vi "Init.vi"(8 "Error In":errorcluster, 11 "Communicator in":refnum<class "Communicator.lvclass">) -> (0 "Error Out":errorcluster, 3 "Communicator out":refnum<class "Communicator.lvclass">)   [LabVIEW 2019, in "Communicator.lvclass"]
uses:
  Communicator.lvclass
  Interfaces/IConfigure/IConfigure.lvclass
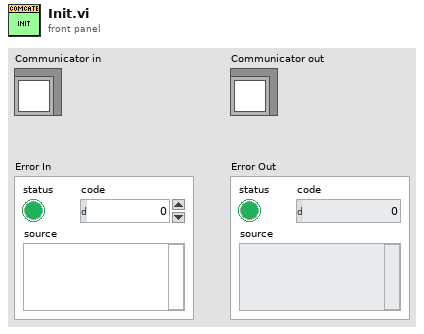
[diagram p1: front panel]
types:
  T1 = typedef "Communicator.lvclass/ObjectAttributes.ctl" = cluster{"IConfigure":refnum<class "IConfigure.lvclass">, "Worker Enqueuer":refnum<class "Message Enqueuer.lvclass">, "Start Counter":i32, "Msg Sent":refnum<user-event>}
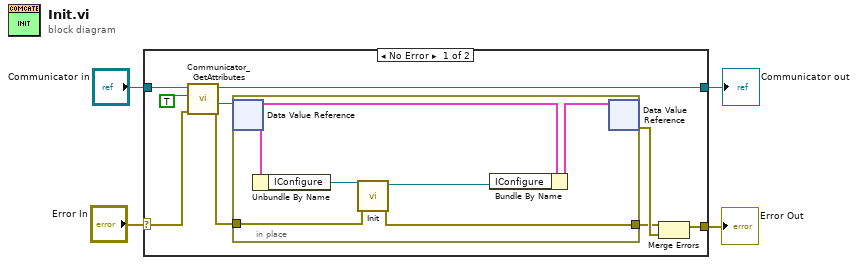
[diagram p0: block diagram]
diagram:
  n1 = case shown="No Error" "Error In" {
    selector: "Error In" -> [w6 w21]
    tunnel: [w11 w21] -> w3
    tunnel: [w12 w20] -> w1
    tunnel: "Communicator in" -> [w5 w20]
    frame No Error {
      n2 = call "Communicator_GetAttributes.vi"("Error In"=w6, "OnlyGetDvrReference(False)"=TRUE, "Communicator in"=w5) -> ("Error Out"=w8:errorcluster, "DataRef"=w10:refnum<data-value>, "Communicator out"=w12:refnum<class "Communicator.lvclass">)  [unwired: 5 in, 1 out]
      n3 = in-place {
        in-place-border: w8 -> [w17]
        in-place-border: [w14] -> w7
        n4 = in-place-dvr #1(w10) -> (w18:T1)  [unwired: 1 out]
        n5 = Unbundle By Name(w18) -> ("IConfigure"=w16:refnum<class "IConfigure.lvclass">)
        n6 = call-dynamic "Init.vi"("error in"=w17, "IInitialize in"=w16) -> ("error out"=w14:errorcluster, "IInitialize out"=w15:refnum<class "IConfigure.lvclass">)  [unwired: 8 in]
        n7 = Bundle By Name(cluster=w18, "IConfigure"=w15) -> (w19:T1)
        n8 = in-place-dvr #1(w19) -> (w13:errorcluster)  [unwired: 1 out]
      }
      n9 = Merge Errors(w7, w13) -> (w11:errorcluster)
    }
    frame Error {
    }
  }
  "Error Out" <- w3
  "Communicator out" <- w1
